vi "Oval 2 Points .vi"(7 "NoOfPoints":u16=100, 9 "IP Results":T1) -> (1 "Y Points":fxp<+/-,20,5>[](array[numeric]), 2 "X Points":fxp<+/-,20,5>[](array[numeric]))   [LabVIEW 2015]
uses:
  IP Dev Area/IP results.ctl
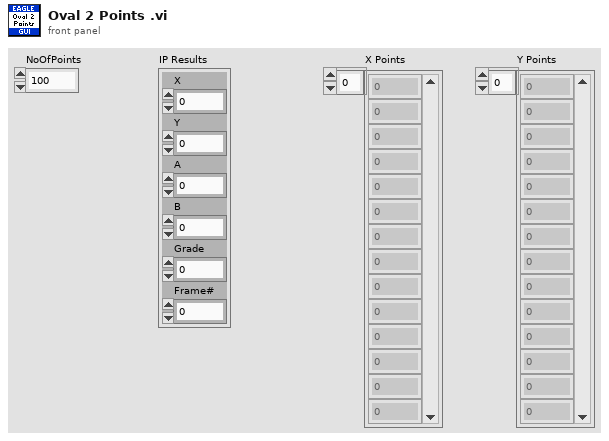
[diagram p1: front panel]
types:
  T1 = typedef "IP results.ctl" = cluster{"X":u16, "Y":u16, "A":dbl, "B":dbl, "Grade":u16, "Frame#":u16}
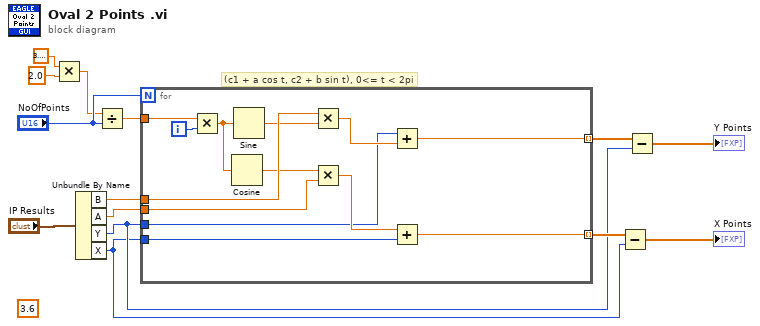
[diagram p0: block diagram]
diagram:
  (unwired) 3.6
  # "(c1 + a cos t, c2 + b sin t), 0<= t < 2pi"
  n1 = Multiply(x=3.141592653589793, y=2.0) -> (x*y=w9:dbl)
  n2 = Unbundle By Name("IP Results") -> ("B"=w6:dbl, "A"=w5:dbl, "Y"=w3:u16, "X"=w1:u16)
  n3 = Divide(x=w9, y="NoOfPoints") -> (x/y=w13:dbl)
  n4 = for {
    N: "NoOfPoints" -> [_]
    tunnel: w3 -> [w24]
    tunnel: w6 -> [w23]
    tunnel: w1 -> [w22]
    tunnel: w5 -> [w21]
    tunnel: w13 -> [w17]
    tunnel: [w15] -> w12 mode=indexing
    tunnel: [w16] -> w7 mode=indexing
    i -> [w20]
    n5 = Multiply(x=w17, y=w20) -> (x*y=w25:dbl)
    n6 = Cosine(x=w25) -> (cos(x)=w18:dbl)
    n7 = Sine(x=w25) -> (sin(x)=w19:dbl)
    n8 = Multiply(x=w23, y=w19) -> (x*y=w27:dbl)
    n9 = Multiply(x=w18, y=w21) -> (x*y=w26:dbl)
    n10 = Add(x=w24, y=w27) -> (x+y=w16:dbl)
    n11 = Add(x=w26, y=w22) -> (x+y=w15:dbl)
  }
  n12 = Subtract(x=w12, y=w1) -> (x-y=→"X Points":dbl[])
  n13 = Subtract(x=w7, y=w3) -> (x-y=→"Y Points":dbl[])
